vi "subProbeEvaluateBreakpointCondition.vi"(10 "String condition":string, 11 "String in":string) -> (2 "Break?":bool, 3 "String":string)   [LabVIEW 2020, in "LabVIEWObjectInterfaces.lvlib" / "ILabVIEWItem.lvclass"]
uses:
  ILabVIEWItem.lvclass
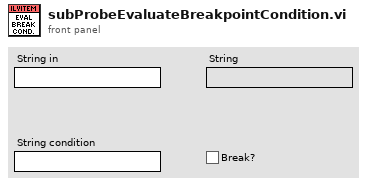
[diagram p1: front panel]
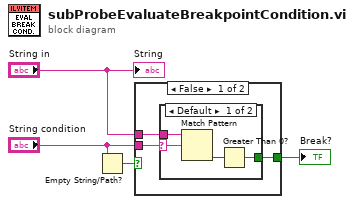
[diagram p0: block diagram]
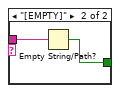
[diagram p2: hidden frame]
diagram:
  n1 = Empty String/Path?(string/path="String condition") -> (empty?=w3:bool)
  n2 = case shown="False" w3 {
    tunnel: "String condition" -> [w7 _]
    tunnel: "String in" -> [w6 _]
    tunnel: [w5 _] -> w4
    frame False {
      n3 = case shown="Default" w7 {
        selector: w7 -> [w11 _]
        tunnel: w6 -> [w10 w13]
        tunnel: [w8 w12] -> w5
        frame Default {
          n4 = Match Pattern(string=w10, regular expression=w11) -> (offset past match=w9:i32)  [unwired: 1 in, 3 out]
          n5 = Greater Than 0?(x=w9) -> (x > 0?=w8:bool)
        }
        frame "[EMPTY]" {
          n6 = Empty String/Path?(string/path=w13) -> (empty?=w12:bool)
        }
      }
    }
    frame True {
    }
  }
  "Break?" <- w4
  "String" <- "String in"
